vi "pracownia7_kulaga.vi"() -> ()   [LabVIEW 2019]
uses:
  <vilib>/Platform/TimedLoop/XDataNode/timing_clust.ctl
  <vilib>/Platform/TimedLoop/XDataNode/nitl_modes.ctl
  <vilib>/Platform/TimedLoop/XDataNode/wakeup.ctl
  <vilib>/Platform/TimedLoop/scheduler/LVUserAPI/_suppVIs/Create_1kHz_TSource.vi
  <vilib>/platform/TimedLoop/XDataNode/XDataNode.xnode
  <vilib>/Platform/TimedLoop/XDataNode/XDNodeRunTimeDep.lvlib
panel:
  in  "Synchronizacja":bool
  out "2":bool
  out "Error 2":errorcluster
  out "L2 Stop":u32
  out "L2 End":i64
  out "Iteracja pêtli 2":i32
  out "L1 Stop":u32
  out "czas_pocz":u32
  out "?":bool
  out "Error 1":errorcluster
  out "S0 End":i64
  out "Iteracja pêtli 1":i64
  out "L1 End":i64
  in  "Okres(s)":dbl min=0.5 max=20.0 step=0.5
  out "S0 Start":i64
  # "1"
  # "TAK"
  # "NIE"
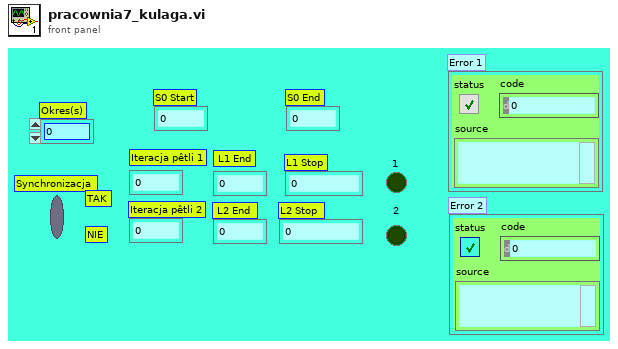
[diagram p1: front panel]
types:
  T1 = typedef "XDNodeRunTimeDep.lvlib/timing_clust.ctl" = cluster{"Expected End [f-1]":u64, "Actual End [f-1]":u64, "Finished Late? [f-1]":bool, "Expected End [i-1]":u64, "Actual End [i-1]":u64, "Finished Late? [i-1]":bool, "Expected Start [i]":u64, "Actual Start [i]":u64, "Expected Start [f]":u64, "Actual Start [f]":u64, "Source Name":string, "Structure Name":string, "Period":i64, "Deadline":i64, "Offset":i64, "Start":i64, "Priority":i32, "Timeout":i32, "Mode":T2, "Wakeup Reason":T3, "Error":errorcluster, "Source Type":string, "Secondary Source Type":string, "Global End Time":u64, "Global Start Time":u64, "Frame Duration":u64, "Iteration Duration":u64, "Assigned CPU":i32, "I/O Scan Engine Mode":u32}
  T2 = typedef "XDNodeRunTimeDep.lvlib/nitl_modes.ctl" = enum32{"No Change", "Process missed periods, maintain original phase", "Discard missed periods, maintain original phase", "Process missed periods, ignore original phase", "Discard missed periods, ignore original phase"}
  T3 = typedef "XDNodeRunTimeDep.lvlib/wakeup.ctl" = enum32{"Normal", "Aborted", "Asynchronous wakeup", "Timing source error", "Timed loop error", "Timeout"}
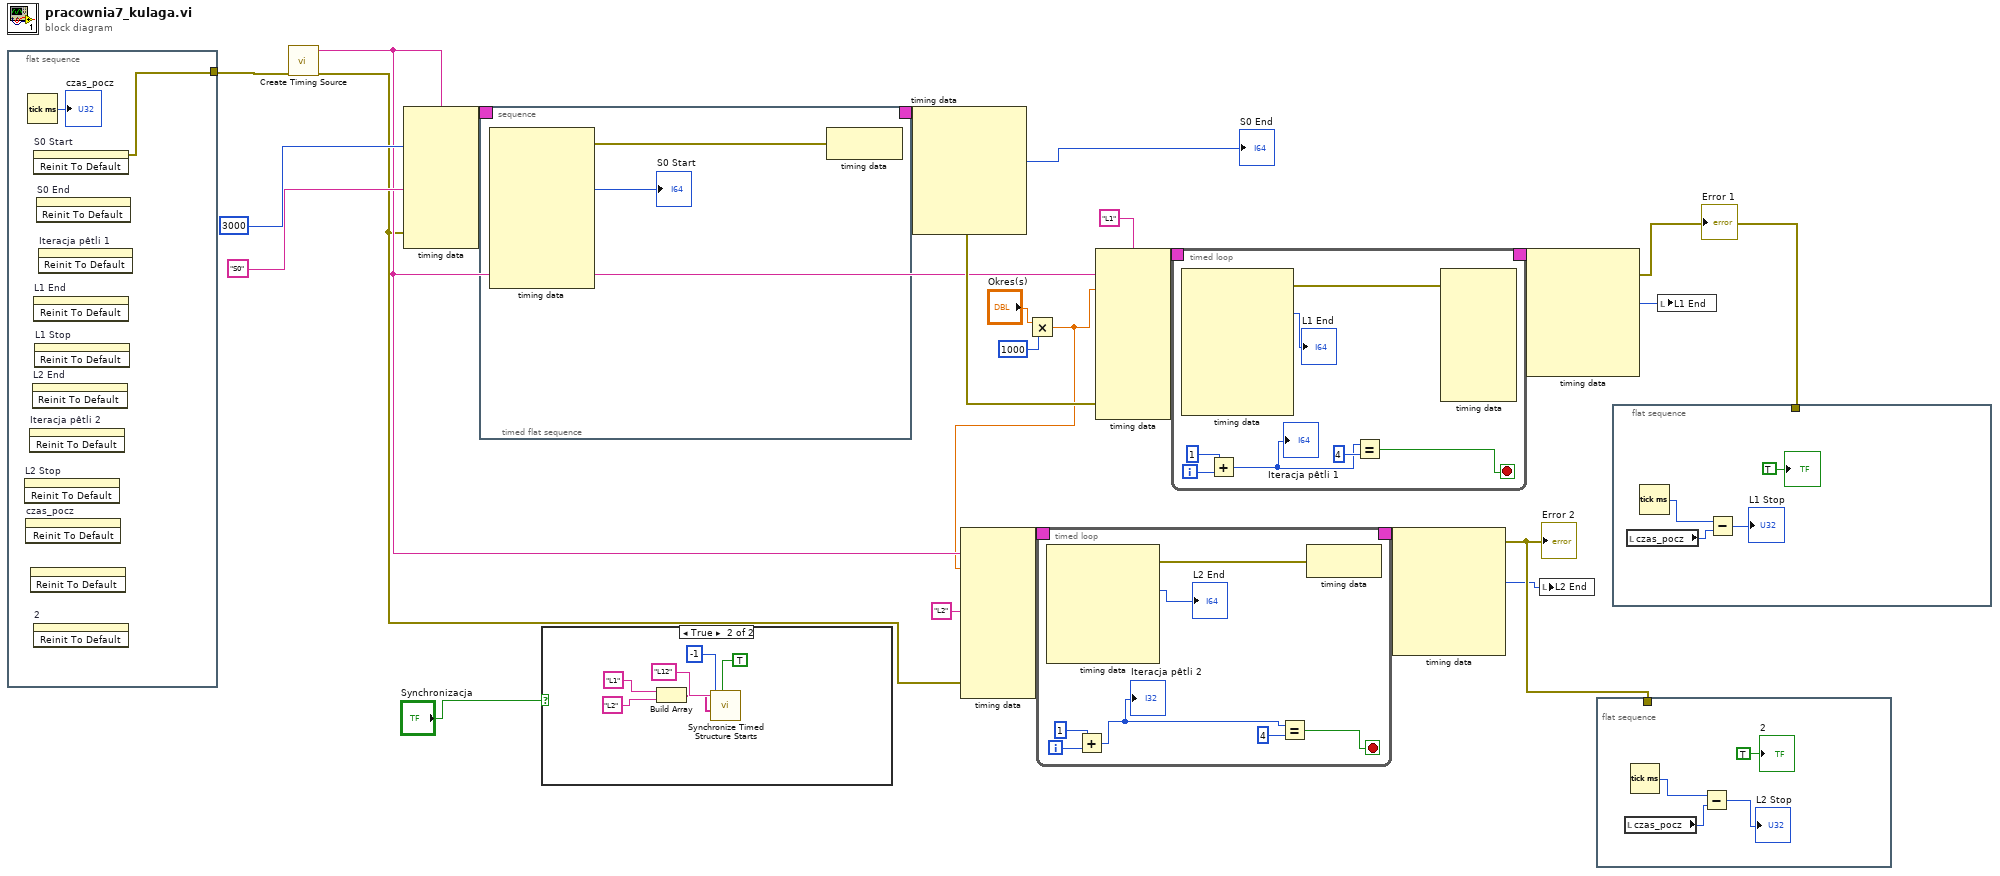
[diagram p0: block diagram]
diagram:
  n1 = flat-sequence {
    tunnel: [w24] -> w2
    frame #0 {
      n2 = invoke on="L2 Stop" class="DigNum (strict)" method="Reinit To Default"() -> ()  [unwired: 3 in, 3 out]
      n3 = invoke on="czas_pocz" class="DigNum (strict)" method="Reinit To Default"() -> ()  [unwired: 3 in, 3 out]
      n4 = Tick Count (ms)() -> (millisecond timer value=→"czas_pocz":u32)
      n5 = invoke on="Iteracja pêtli 2" class="DigNum (strict)" method="Reinit To Default"() -> ()  [unwired: 3 in, 3 out]
      n6 = invoke class="Bool (strict)" method="Reinit To Default"() -> ()  [unwired: 3 in, 3 out]
      n7 = invoke on="L2 End" class="DigNum (strict)" method="Reinit To Default"() -> ()  [unwired: 3 in, 3 out]
      n8 = invoke on="S0 Start" class="DigNum (strict)" method="Reinit To Default"() -> (error out=w24:errorcluster)  [unwired: 3 in, 2 out]
      n9 = invoke on="L1 End" class="DigNum (strict)" method="Reinit To Default"() -> ()  [unwired: 3 in, 3 out]
      n10 = invoke on="2" class="Bool (strict)" method="Reinit To Default"() -> ()  [unwired: 3 in, 3 out]
      n11 = invoke on="L1 Stop" class="DigNum (strict)" method="Reinit To Default"() -> ()  [unwired: 3 in, 3 out]
      n12 = invoke on="S0 End" class="DigNum (strict)" method="Reinit To Default"() -> ()  [unwired: 3 in, 3 out]
      n13 = invoke on="Iteracja pêtli 1" class="DigNum (strict)" method="Reinit To Default"() -> ()  [unwired: 3 in, 3 out]
    }
  }
  n14 = call-poly <vilib>:"Create Timing Source.vi"("error in (no error)"=w2) -> ("error out"=w4:errorcluster, "name (out)"=w9:string)  [unwired: 9 in]
  n15 = node-c288(w9, i64 3000 ("Offset"), "S0" ("Structure Name"), w4) -> (w19:T1)  [unwired: 4 in]
  n16 = timed-sequence {
    timing: w19 -> [_]
    timing-out: [_] -> w18
    n17 = timed-flat-sequence {
      n18 = node-c288() -> (w26:errorcluster, →"S0 Start":i64)  [unwired: 1 in, 8 out]
      n19 = node-c288(w26) -> ()  [unwired: 1 out]
    }
  }
  n20 = case shown="True" "Synchronizacja" {
    frame False {
    }
    frame True {
      n21 = Build Array("L1" ("Structure Name"), "L2" ("Structure Name")) -> (w35:string[])
      n22 = call <vilib>:"Synchronize Timed Structure Starts.vi"("replace (T)"=TRUE, "timed structure names"=w35, "timeout ms (10000)"=-1, "synchronization group name"="L12") -> ()  [unwired: 6 in, 2 out]
    }
  }
  n23 = node-c288(w18) -> (w17:errorcluster, →"S0 End":i64)  [unwired: 5 out]
  n24 = Multiply(x="Okres(s)", y=i64 1000) -> (x*y=w5:dbl)
  n25 = node-c288(w9, w5, "L2" ("Structure Name"), w4) -> (w21:T1)  [unwired: 6 in]
  n26 = timed-loop {
    timing: w21 -> [_]
    timing-out: [_] -> w20
    i -> [w46]
    stop <- w43 stop-if-true
    n27 = node-c288() -> (w40:errorcluster, →"L2 End":i64)  [unwired: 1 in, 5 out]
    n28 = Add(x=1, y=w46) -> (x+y=w42:i32)
    "Iteracja pêtli 2" <- w42
    n29 = Equal?(x=w42, y=4) -> (x = y?=w43:bool)
    n30 = node-c288(w40) -> ()  [unwired: 1 out]
  }
  n31 = node-c288(w9, w5, "L1" ("Structure Name"), w17) -> (w23:T1)  [unwired: 6 in]
  n32 = timed-loop {
    timing: w23 -> [_]
    timing-out: [_] -> w22
    i -> [w56]
    stop <- w57 stop-if-true
    n33 = node-c288() -> (w53:errorcluster, →"L1 End":i64)  [unwired: 1 in, 7 out]
    n34 = Add(x=1, y=w56) -> (x+y=w54:i32)
    "Iteracja pêtli 1" <- w54
    n35 = Equal?(x=w54, y=4) -> (x = y?=w57:bool)
    n36 = node-c288(w53) -> ()  [unwired: 7 in, 1 out]
  }
  n37 = node-c288(w20) -> (w8:errorcluster, w3:i64)  [unwired: 5 out]
  "Error 2" <- w8
  n38 = node-c288(w22) -> (w16:errorcluster, w12:i64)  [unwired: 5 out]
  "Error 1" <- w16
  n39 = local write "L2 End"(w3) -> ()
  n40 = flat-sequence {
    tunnel: w8 -> [_]
    frame #0 {
      n41 = local read "czas_pocz"() -> (w67:u32)
      n42 = Tick Count (ms)() -> (millisecond timer value=w68:u32)
      n43 = Subtract(x=w68, y=w67) -> (x-y=→"L2 Stop":u32)
      "2" <- TRUE ("Boolean 2")
    }
  }
  n44 = flat-sequence {
    tunnel: w16 -> [_]
    frame #0 {
      n45 = local read "czas_pocz"() -> (w70:u32)
      n46 = Tick Count (ms)() -> (millisecond timer value=w71:u32)
      n47 = Subtract(x=w71, y=w70) -> (x-y=→"L1 Stop":u32)
      "?" <- TRUE ("Boolean1")
    }
  }
  n48 = local write "L1 End"(w12) -> ()
